vi "medicaoIXV.vi"() -> ()   [LabVIEW 2012]
uses:
  <vilib>/Utility/file.llb/Write To Spreadsheet File (string).vi
  <vilib>/Utility/file.llb/Write To Spreadsheet File (DBL).vi
  <instrlib>/Agilent 6XXX Series/Agilent 6XXX Series.lvlib
panel:
  out "array":dbl[][](array[numeric])
  in  "Tab Control":enum32{"Entrada de dados", "Saída de dados"}(tab)
  out "ON/OFF":bool
  in  "Pontos":dbl
  in  "Tensão máxima":dbl
  in  "Nome da célula":string
  in  "Local":path
  in  "Delay(s)":dbl
  in  "Start":bool
  in  "Print Screen":bool
  out "IXV":cluster{"Y":dbl[], "Y":dbl[]}[](graph)
  out "output voltage":dbl
  out "Tensao Atual":dbl
  out "Corrente Atual":dbl
  out "Ponto Atual":i32
  out "TABELA DE DADOS\nTensão(fonte)     Tensão                  Corrente            Pontos":dbl[][](array[numeric]) caption="all rows" format="%0.3f"
  in  "stop":bool
  in  "CorrenteGraph":dbl
  in  "error in (no error)":errorcluster
  out "error out":errorcluster
  in  "TensaoGraph":dbl
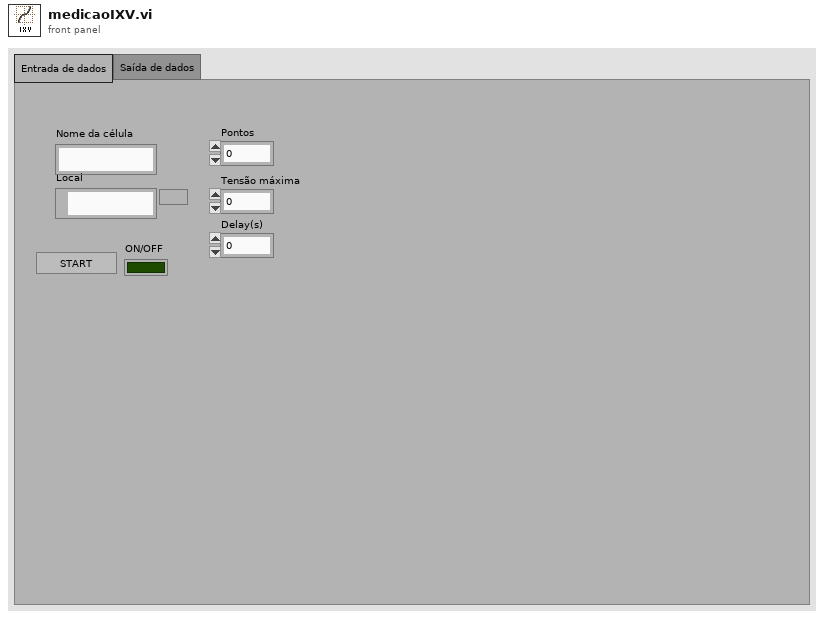
[diagram p1: front panel]
types:
  T1 = typedef "imagedata.ctl" = cluster{"image type":i32, "image depth":i32, "image":u8[], "mask":u8[], "colors":u32[], "Rectangle":cluster{"left":i16, "top":i16, "right":i16, "bottom":i16}}
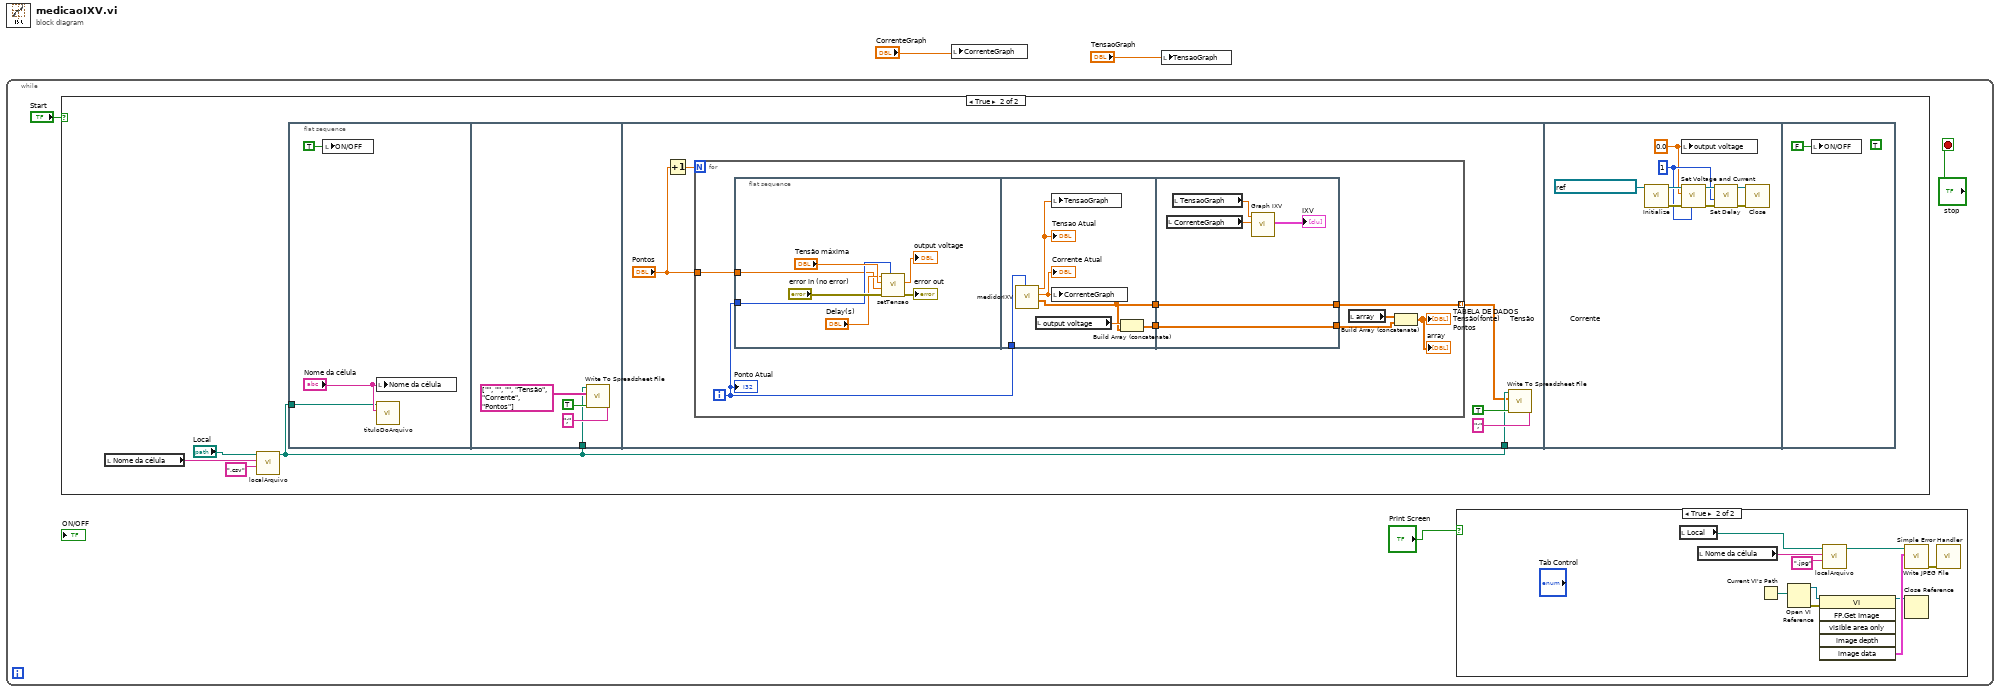
[diagram p0: block diagram]
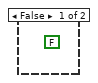
[diagram p3: hidden frame]
diagram:
  n1 = while {
    stop <- "stop" stop-if-true
    n2 = case shown="True" "Start" {
      frame False {
        (unwired) FALSE
      }
      frame True {
        n3 = local read "Nome da célula"() -> (w16:string)
        n4 = call "localArquivo.vi"("extensão"=".csv", "Nome do arquivo"=w16, "Local"="Local") -> ("Path"=w18:path)  [unwired: 8 in]
        n5 = flat-sequence {
          tunnel: w18 -> [w21]
          tunnel: w18 -> [w23]
          tunnel: w18 -> [w30]
          frame #0 {
            n6 = local write "ON/OFF"(TRUE ("ON/OFF")) -> ()
            n7 = local write "Nome da célula"("Nome da célula") -> ()
            n8 = call "tituloDoArquivo.vi"("Nome da célula"="Nome da célula", "file path (dialog if empty)"=w21) -> ()  [unwired: 10 in]
          }
          frame #1 {
            n9 = call-poly <vilib>:"Write To Spreadsheet File.vi"("delimiter (\\t)"=";" ("delimiter (\\t)"), "append to file? (new file:F)"=TRUE, "2D data"=string[][] [["", "", ""], ["Tensão", "Corrente", "Pontos"]], "file path (dialog if empty)"=w23) -> ()  [unwired: 4 in, 1 out]
          }
          frame #2 {
            n10 = Increment(x="Pontos") -> (x+1=w29:dbl)
            n11 = for {
              N: w29 -> [_]
              tunnel: [w38] -> w27 mode=indexing
              tunnel: "Pontos" -> [w40]
              i -> [w39]
              n12 = flat-sequence {
                tunnel: w40 -> [w43]
                tunnel: w39 -> [w44]
                tunnel: w39 -> [w53]
                tunnel: [w48] -> w37
                tunnel: [w50] -> w36
                tunnel: [w57] -> w35
                tunnel: [w58] -> w38
                tunnel: w37 -> [w58]
                tunnel: w36 -> [w57]
                frame #0 {
                  n13 = call "setTensao.vi"("Ponto"=w44, "error in (no error)"="error in (no error)", "Pontos"=w43, "Tensão máxima"="Tensão máxima", "delay(s)"="Delay(s)") -> ("error out"=→"error out":errorcluster, "output voltage"=→"output voltage":dbl)  [unwired: 5 in]
                }
                frame #1 {
                  n14 = call "medidorIXV.vi"("Ponto"=w53) -> ("Array"=w48:dbl[], "Corrente Atual"=w52:dbl, "Tensao Atual"=w51:dbl)  [unwired: 8 in]
                  "Corrente Atual" <- w52
                  "Tensao Atual" <- w51
                  n15 = local read "output voltage"() -> (w49:dbl)
                  n16 = local write "TensaoGraph"(w51) -> ()
                  n17 = local write "CorrenteGraph"(w52) -> ()
                  n18 = Build Array (concatenate)(w49, w48) -> (w50:dbl[])
                }
                frame #2 {
                  n19 = local read "CorrenteGraph"() -> (w54:dbl)
                  n20 = local read "TensaoGraph"() -> (w55:dbl)
                  n21 = call "Graph IXV"("Y Input"=w54, "X Input"=w55) -> ("XY Graph"=→"IXV":cluster{"Y":dbl[], "Y":dbl[]}[])  [unwired: 3 in, 6 out]
                }
              }
              n22 = local read "array"() -> (w34:dbl[][])
              n23 = Build Array (concatenate)(w34, w35) -> (→"TABELA DE DADOS\nTensão(fonte)     Tensão                  Corrente            Pontos" →"array":dbl[][])
              "Ponto Atual" <- w39
            }
            n24 = call-poly <vilib>:"Write To Spreadsheet File.vi"("delimiter (\\t)"=";" ("delimiter (\\t)"), "append to file? (new file:F)"=TRUE, "2D data"=w27, "file path (dialog if empty)"=w30) -> ()  [unwired: 4 in, 1 out]
          }
          frame #3 {
            w59 = 0.0 ("voltage (0 V)")
            w62 = u8 1 ("channel (1)")
            n25 = call <instrlib>:"Initialize.vi"("VISA resource name"=refnum<visa-resource-name> "GPIB0::5::INSTR") -> ("error out"=w64:errorcluster, "VISA resource name out"=w63:refnum<visa-resource-name>)  [unwired: 9 in]
            n26 = local write "output voltage"(w59) -> ()
            n27 = call <instrlib>:"Set Voltage and Current.vi"("channel (1)"=w62, "error in (no error)"=w64, "voltage (0 V)"=w59, "VISA resource name"=w63) -> ("error out"=w65:errorcluster, "VISA resource name out"=w66:refnum<visa-resource-name>)  [unwired: 6 in]
            n28 = call <instrlib>:"Set Delay.vi"("error in (no error)"=w65, "channel (1)"=w62, "VISA resource name"=w66) -> ("error out"=w60:errorcluster, "VISA resource name out"=w61:refnum<visa-resource-name>)  [unwired: 7 in]
            n29 = call <instrlib>:"Close.vi"("error in (no error)"=w60, "VISA resource name"=w61) -> ()  [unwired: 9 in, 1 out]
          }
          frame #4 {
            (unwired) TRUE
            n30 = local write "ON/OFF"(FALSE) -> ()
          }
        }
      }
    }
    n31 = case shown="True" "Print Screen" {
      frame False {
      }
      frame True {
        n32 = local read "Local"() -> (w14:path)
        n33 = local read "Nome da célula"() -> (w15:string)
        n34 = Current VI's Path() -> (path=w9:path)
        n35 = Open VI Reference(vi path=w9) -> (vi reference=w8:refnum<vi>, error out=w7:errorcluster)  [unwired: 5 in]
        n36 = invoke class="VI" method="FP.Get Image"(reference=w8, error in=w7) -> (reference out=w10:refnum<vi>, "image data"=w11:T1)  [unwired: 4 in, 4 out]
        n37 = call "localArquivo.vi"("extensão"=".jpg", "Nome do arquivo"=w15, "Local"=w14) -> ("Path"=w6:path)  [unwired: 8 in]
        n38 = call <vilib>:"Write JPEG File.vi"("image data"=w11, "path to JPEG file"=w6) -> ("error out"=w12:errorcluster)  [unwired: 8 in, 1 out]
        n39 = Close Reference(reference=w10) -> ()  [unwired: 1 in, 1 out]
        n40 = call <vilib>:"Simple Error Handler.vi"("error in (no error)"=w12) -> ()  [unwired: 4 in, 5 out]
      }
    }
  }
  n41 = local write "CorrenteGraph"("CorrenteGraph") -> ()
  n42 = local write "TensaoGraph"("TensaoGraph") -> ()
